vi "json_test-error.vi"(7 "indent level":i32, 10 "error":errorcluster) -> (2 "indented string":string)   [LabVIEW 2013, in "Caraya.lvlib" / "Test Result.lvclass"]
uses:
  Test Result.lvclass
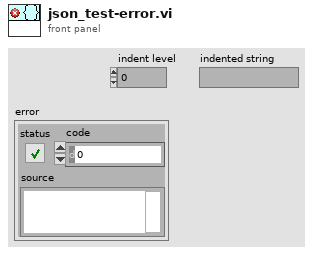
[diagram p1: front panel]
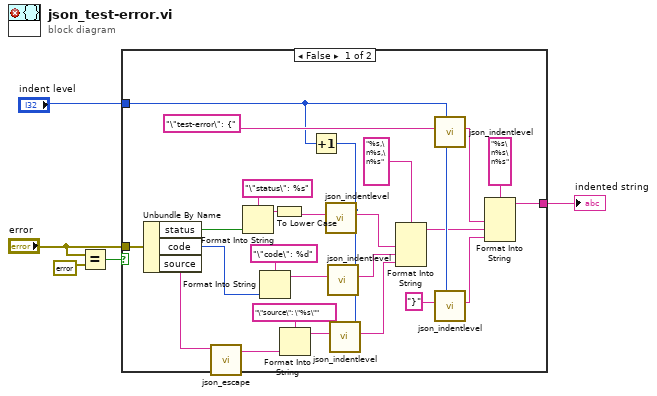
[diagram p0: block diagram]
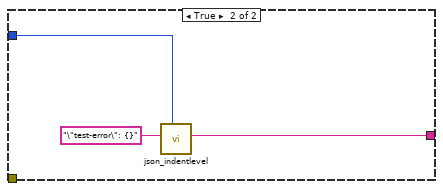
[diagram p2: hidden frame]
diagram:
  n1 = Equal?(x="error", y=errorcluster {"status"=FALSE, "code"=0, "source"=""}) -> (x = y?=w3:bool)
  n2 = case shown="False" w3 {
    tunnel: "error" -> [w30 _]
    tunnel: [w25 w32] -> w1
    tunnel: "indent level" -> [w19 w31]
    frame False {
      n3 = Unbundle By Name(w30) -> ("status"=w21:bool, "code"=w15:i32, "source"=w13:string)
      n4 = call "json_escape.vi"("string"=w13) -> ("escaped string"=w12:string)  [unwired: 10 in]
      n5 = Format Into String(format string="\"status\": %s", w21) -> (resulting string=w22:string)  [unwired: 2 in, 1 out]
      n6 = Format Into String(format string="\"code\": %d", w15) -> (resulting string=w6:string)  [unwired: 2 in, 1 out]
      n7 = To Lower Case(string=w22) -> (all lower case string=w20:string)
      n8 = Format Into String(format string="\"source\": \"%s\"", w12) -> (resulting string=w10:string)  [unwired: 2 in, 1 out]
      n9 = Increment(x=w19) -> (x+1=w9:i32)
      n10 = call "json_indentlevel.vi"("indent level"=w9, "string"=w20) -> ("indented string"=w18:string)  [unwired: 9 in]
      n11 = call "json_indentlevel.vi"("indent level"=w9, "string"=w6) -> ("indented string"=w14:string)  [unwired: 9 in]
      n12 = call "json_indentlevel.vi"("indent level"=w9, "string"=w10) -> ("indented string"=w8:string)  [unwired: 9 in]
      n13 = Format Into String(format string="%s,\n%s,\n%s", w18, w14, w8) -> (resulting string=w7:string)  [unwired: 2 in, 1 out]
      n14 = call "json_indentlevel.vi"("indent level"=w19, "string"="\"test-error\": {" ("JSON string")) -> ("indented string"=w27:string)  [unwired: 9 in]
      n15 = call "json_indentlevel.vi"("indent level"=w19, "string"="}") -> ("indented string"=w26:string)  [unwired: 9 in]
      n16 = Format Into String(format string="%s\n%s\n%s", w27, w7, w26) -> (resulting string=w25:string)  [unwired: 2 in, 1 out]
    }
    frame True {
      n17 = call "json_indentlevel.vi"("indent level"=w31, "string"="\"test-error\": {}" ("JSON string")) -> ("indented string"=w32:string)  [unwired: 9 in]
    }
  }
  "indented string" <- w1
